vi "Display Table.vi"(0 "Listbox":refnum<vi>, 5 "Table Items":string[][](array[string]), 7 "Properties":T3, 9 "Columns":T1[](array[typedef]), 11 "error in (no error)":errorcluster) -> (4 "reference out":refnum<vi>, 15 "error out":errorcluster)   [LabVIEW 2020, in "KTable.xctl"]
uses:
  KTable.xctl
  Table Properties.ctl
  ColumnSpec.ctl
  ColumnType.ctl
  <vilib>/Utility/miscctls.llb/LVRowAndColumnTypeDef.ctl
  Array Manipulation VIs/Array-Dimensions (2D string).vi
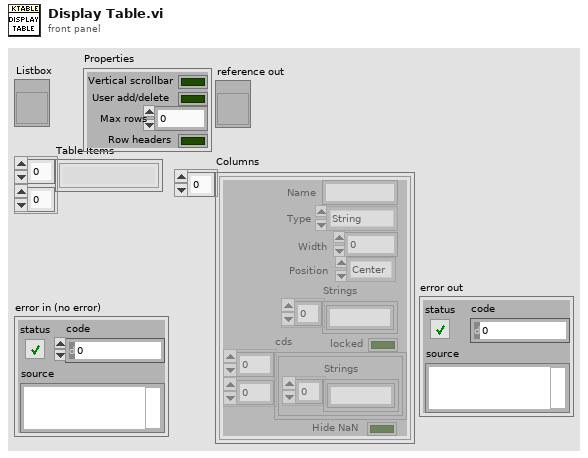
[diagram p1: front panel]
types:
  T1 = typedef "KTable.xctl/ColumnSpec.ctl" = cluster{"Name":string, "Type":T2, "Width":i32, "Strings":string[], "Position":enum16{"Left", "Center", "Right"}, "locked":bool, "cds":cluster{"Strings":string[]}[][], "Hide NaN":bool}
  T2 = typedef "KTable.xctl/ColumnType.ctl" = enum16{"String", "Enum", "Int", "Double", "Boolean", "Ring", "Formula", "Color"}
  T3 = typedef "KTable.xctl/Table Properties.ctl" = cluster{"Vertical scrollbar":bool, "User add/delete":bool, "Max rows":i32, "Row headers":bool}
  T4 = typedef "LVRowAndColumnTypeDef.ctl" = cluster{"Row":i32, "Column":i32}
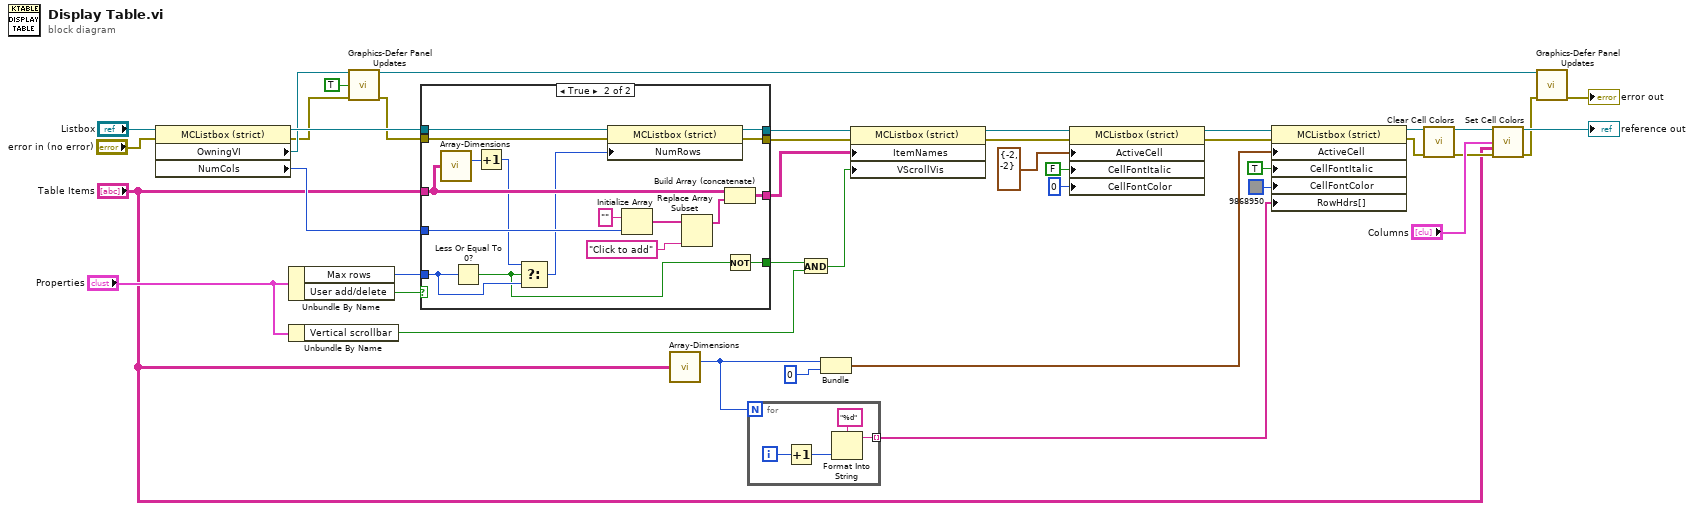
[diagram p0: block diagram]
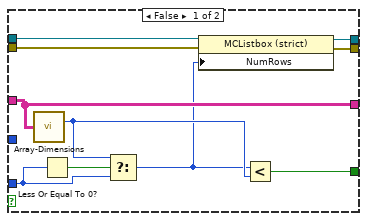
[diagram p2: hidden frame]
diagram:
  n1 = property class="MCListbox (strict)"(reference="Listbox", error in="error in (no error)") -> (reference out=w30:refnum<vi>, error out=w13:errorcluster, "OwningVI"=w14:refnum<vi>, "NumCols"=w15:u32)
  n2 = Unbundle By Name("Properties") -> ("Max rows"=w26:i32, "User add/delete"=w27:bool)
  n3 = Unbundle By Name("Properties") -> ("Vertical scrollbar"=w24:bool)
  n4 = call "Graphics-Defer Panel Updates.vi"("VI"=w14, "Defer (F)"=TRUE, "error in (no error)"=w13) -> ("VI out"=w11:refnum<vi>, "error out"=w12:errorcluster)  [unwired: 11 in]
  n5 = case shown="True" w27 {
    tunnel: "Table Items" -> [w46 w59]
    tunnel: [w46 w67] -> w21
    tunnel: w15 -> [_ w57]
    tunnel: w30 -> [w50 w63]
    tunnel: w12 -> [w47 w62]
    tunnel: [w49 w61] -> w29
    tunnel: [w48 w60] -> w28
    tunnel: w26 -> [w44 w55]
    tunnel: [w42 w53] -> w22
    frame False {
      n6 = call-poly "Array-Dimensions.vi"("2D Array"=w46) -> ("# rows"=w43:i32)  [unwired: 13 in, 1 out]
      n7 = Less Or Equal To 0?(x=w44) -> (x <= 0?=w45:bool)
      n8 = Select(t=w43, s=w45, f=w44) -> (s? t:f=w41:i32)
      n9 = property class="MCListbox (strict)"(reference=w50, error in=w47, "NumRows"=w41) -> (reference out=w49:refnum<vi>, error out=w48:errorcluster)
      n10 = Less?(x=w41, y=w43) -> (x < y?=w42:bool)
    }
    frame True {
      n11 = call-poly "Array-Dimensions.vi"("2D Array"=w59) -> ("# rows"=w58:i32)  [unwired: 13 in, 1 out]
      n12 = Less Or Equal To 0?(x=w55) -> (x <= 0?=w52:bool)
      n13 = Increment(x=w58) -> (x+1=w54:i32)
      n14 = Select(t=w54, s=w52, f=w55) -> (s? t:f=w51:i32)
      n15 = property class="MCListbox (strict)"(reference=w63, error in=w62, "NumRows"=w51) -> (reference out=w61:refnum<vi>, error out=w60:errorcluster)
      n16 = Initialize Array("" ("element"), w57) -> (w66:string[])
      n17 = Replace Array Subset(array=w66, new element="Click to add" ("new element/subarray")) -> (w64:string[])  [unwired: 1 in]
      n18 = Build Array (concatenate)(w59, w64) -> (w67:string[][])
      n19 = Not(x=w52) -> (.not. x?=w53:bool)
    }
  }
  n20 = call-poly "Array-Dimensions.vi"("2D Array"="Table Items") -> ("# rows"=w20:i32)  [unwired: 13 in, 1 out]
  n21 = for {
    N: w20 -> [_]
    tunnel: [w69] -> w19 mode=indexing
    i -> [w71]
    n22 = Increment(x=w71) -> (x+1=w68:i32)
    n23 = Format Into String(format string="%d", w68) -> (resulting string=w69:string)  [unwired: 2 in, 1 out]
  }
  n24 = And(x=w22, y=w24) -> (x .and. y?=w23:bool)
  n25 = Bundle("# rows"=w20, 0) -> (w33:cluster{"# rows":i32, i32})  [unwired: 1 in]
  n26 = property class="MCListbox (strict)"(reference=w29, error in=w28, "ItemNames"=w21, "VScrollVis"=w23) -> (reference out=w40:refnum<vi>, error out=w39:errorcluster)
  n27 = property class="MCListbox (strict)"(reference=w40, error in=w39, "ActiveCell"=T4 {"Row"=-2, "Column"=-2} ("Active Cell:Active Cell"), "CellFontItalic"=FALSE ("Active Cell:Cell Font:Italic"), "CellFontColor"=u32 0 ("Active Cell:Cell Font:Color")) -> (reference out=w18:refnum<vi>, error out=w17:errorcluster)
  n28 = property class="MCListbox (strict)"(reference=w18, error in=w17, "ActiveCell"=w33, "CellFontItalic"=TRUE ("Active Cell:Cell Font:Italic"), "CellFontColor"=u32 9868950, "RowHdrs[]"=w19) -> (reference out=w9:refnum<vi>, error out=w8:errorcluster)
  n29 = call "Clear Cell Colors.vi"("MulticolumnListbox in"=w9, "error in (no error)"=w8) -> ("MulticolumnListbox out"=w6:refnum<vi>, "error out"=w5:errorcluster)  [unwired: 12 in]
  n30 = call "Set Cell Colors.vi"("MulticolumnListbox in"=w6, "Columns"="Columns", "Table Items"="Table Items", "error in (no error)"=w5) -> ("MulticolumnListbox out"=→"reference out":refnum<vi>, "error out"=w3:errorcluster)  [unwired: 10 in]
  n31 = call "Graphics-Defer Panel Updates.vi"("VI"=w11, "error in (no error)"=w3) -> ("error out"=→"error out":errorcluster)  [unwired: 12 in, 1 out]
